vi "Sparse FFT.vi"(2 "number of FFT values":i32=1, 3 "X":cdb[](array[numeric]) format="%.2f") -> (0 "error":i32, 1 "FFT {X}":cdb[](array[numeric]) format="%.2f")   [LabVIEW 2018, in "NI_Gmath.lvlib"]
doc: "Computes the first elements of the Fourier transform of the input signal X faster than the FFT."
uses:
  NI_Gmath.lvlib
  Complex FFT.vi
  <vilib>/Analysis/NI_AALPro.lvlib
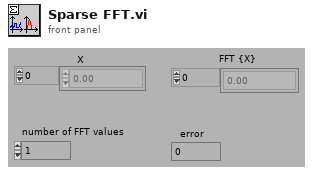
[diagram p1: front panel]
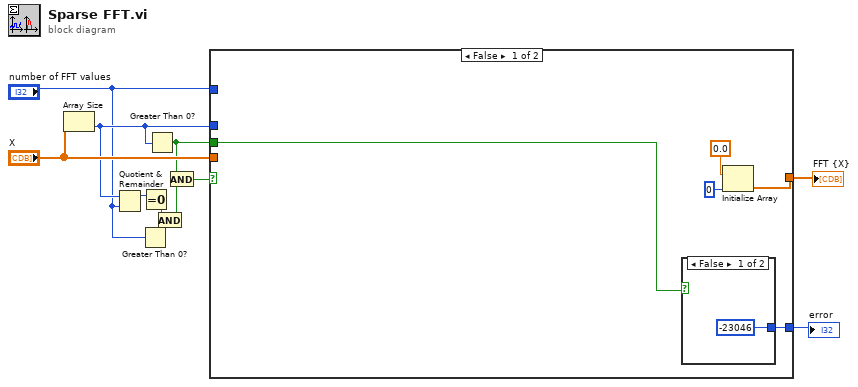
[diagram p0: block diagram]
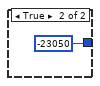
[diagram p2: hidden frame]
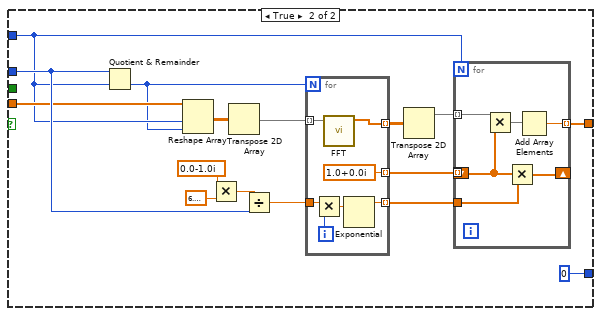
[diagram p3: hidden frame]
diagram:
  n1 = Array Size(array="X") -> (size(s)=w7:i32)
  n2 = Quotient & Remainder(x=w7, y="number of FFT values") -> (x-y*floor(x/y)=w8:i32)  [unwired: 1 out]
  n3 = Greater Than 0?(x="number of FFT values") -> (x > 0?=w2:bool)
  n4 = Equal To 0?(x=w8) -> (x = 0?=w3:bool)
  n5 = Greater Than 0?(x=w7) -> (x > 0?=w5:bool)
  n6 = And(x=w3, y=w2) -> (x .and. y?=w1:bool)
  n7 = And(x=w5, y=w1) -> (x .and. y?=w6:bool)
  n8 = case shown="False" w6 {
    tunnel: w7 -> [_ w33]
    tunnel: "X" -> [_ w32]
    tunnel: "number of FFT values" -> [_ w31]
    tunnel: [w14 w30] -> w11
    tunnel: [w12 0] -> w9
    tunnel: w5 -> [w13 _]
    frame False {
      n9 = case shown="False" w13 {
        tunnel: [-23046 -23050] -> w12
        frame False {
        }
        frame True {
        }
      }
      n10 = Initialize Array(0.0, 0) -> (w14:dbl[])
    }
    frame True {
      n11 = Quotient & Remainder(x=w33, y=w31) -> (floor(x/y)=w29:i32)  [unwired: 1 out]
      n12 = Reshape Array(w32, w31, w29) -> (w28:cdb[][])
      n13 = Multiply(x=cdb 0.0-1.0i, y=6.283185307179586) -> (x*y=w22:cdb)
      n14 = Transpose 2D Array(2D array=w28) -> (transposed array=w27:cdb[][])
      n15 = Divide(x=w22, y=w33) -> (x/y=w23:cdb)
      n16 = for {
        N: w29 -> [_]
        tunnel: w27 -> [w47] mode=indexing
        tunnel: [w46] -> w26 mode=indexing
        tunnel: [cdb 1.0+0.0i] -> w24 mode=indexing
        tunnel: w23 -> [w44]
        tunnel: [w41] -> w34 mode=indexing
        i -> [w43]
        n17 = Multiply(x=w44, y=w43) -> (x*y=w42:cdb)
        n18 = call-poly "FFT.vi"("X"=w47) -> ("FFT {X}"=w46:cdb[])  [unwired: 9 in, 1 out]
        n19 = Exponential(1:w42) -> (0:w41:cdb)
      }
      n20 = Transpose 2D Array(2D array=w26) -> (transposed array=w25:cdb[][])
      n21 = for {
        N: w31 -> [_]
        tunnel: w25 -> [w40] mode=indexing
        tunnel: [w38] -> w30 mode=indexing
        shift-right: [w37] -> _
        shift-left: w24 -> [w36]
        tunnel: [w36] -> _ mode=indexing
        tunnel: w34 -> [w35]
        n22 = Multiply(x=w40, y=w36) -> (x*y=w39:cdb[])
        n23 = Multiply(x=w36, y=w35) -> (x*y=w37:cdb[])
        n24 = Add Array Elements(numeric array=w39) -> (sum=w38:cdb)
      }
    }
  }
  "FFT {X}" <- w11
  "error" <- w9
